vi "Update Dirty Dot Image.vi"(8 "error in (no error)":errorcluster, 10 "Dirty Dot State":bool, 11 "Test Executive Builder Dirty Dot View in":refnum<class "Test Executive Builder Dirty Dot View.lvclass">) -> (0 "error out":errorcluster, 3 "Test Executive Builder Dirty Dot View out":refnum<class "Test Executive Builder Dirty Dot View.lvclass">)   [LabVIEW 2017, in "Test Executive Builder Dirty Dot View.lvclass"]
uses:
  <vilib>/gpm_packages/@cs/Test-executive-builder/Source/Dirty Dot View/Test Executive Builder Dirty Dot View/Test Executive Builder Dirty Dot View.lvclass
  <vilib>/gpm_packages/@cs/Test-executive-builder/Source/Dirty Dot View/Test Executive Builder Dirty Dot View/Test Executive Builder Dirty Dot View.lvclass/Test Executive Builder Dirty Dot View.ctl
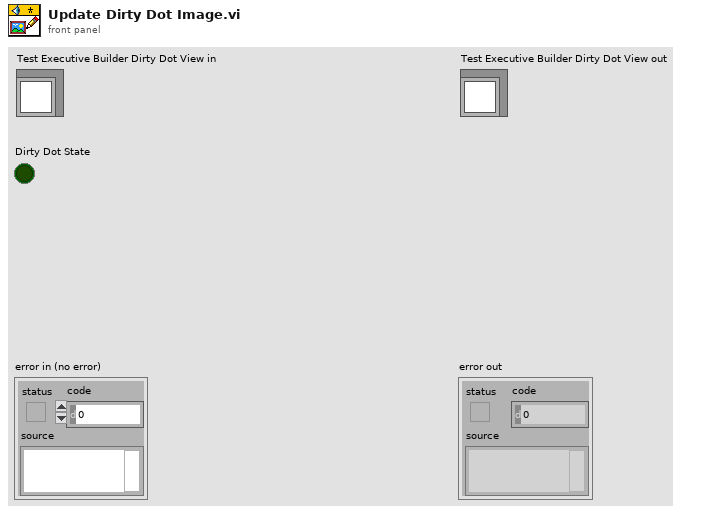
[diagram p1: front panel]
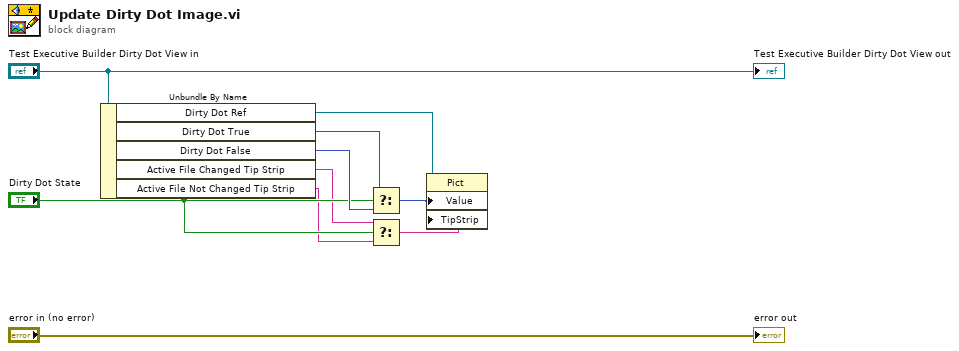
[diagram p0: block diagram]
diagram:
  n1 = Unbundle By Name("Test Executive Builder Dirty Dot View in") -> ("Dirty Dot Ref"=w6:refnum<vi>, "Dirty Dot True"=w7:picture, "Dirty Dot False"=w8:picture, "Active File Changed Tip Strip"=w3:string, "Active File Not Changed Tip Strip"=w2:string)
  n2 = Select(t=w7, s="Dirty Dot State", f=w8) -> (s? t:f=w5:picture)
  n3 = Select(t=w3, s="Dirty Dot State", f=w2) -> (s? t:f=w1:string)
  n4 = property class="Pict"(reference=w6, "Value"=w5, "TipStrip"=w1) -> ()  [unwired: 1 in, 2 out]
  "error out" <- "error in (no error)"
  "Test Executive Builder Dirty Dot View out" <- "Test Executive Builder Dirty Dot View in"
